vi "Create.vi"(8 "error in (no error)":errorcluster, 10 "Selected Group":T1, 11 "Chassis Link":T3) -> (0 "error out":errorcluster, 3 "Preview out":refnum<class "Preview.lvclass">)   [LabVIEW 2012, in "Preview Window.lvlib" / "Preview.lvclass"]
uses:
  Preview.lvclass
  Custom Ctrls/Master Cfg/ge_Cfg wChassis.ctl
  Cfg Grandmaster/Class Chassis BOM/Chassis BOM.lvclass
  Cfg Grandmaster/Class Chassis Cfg/ChassisCfg.lvclass
  Data Acquisition/Class Chassis Tasks/Chassis Tasks.lvclass
  Common/Controls/Selected Group.ctl
  Common/Controls/TE_Designator.ctl
  Preview.lvclass/Preview.ctl
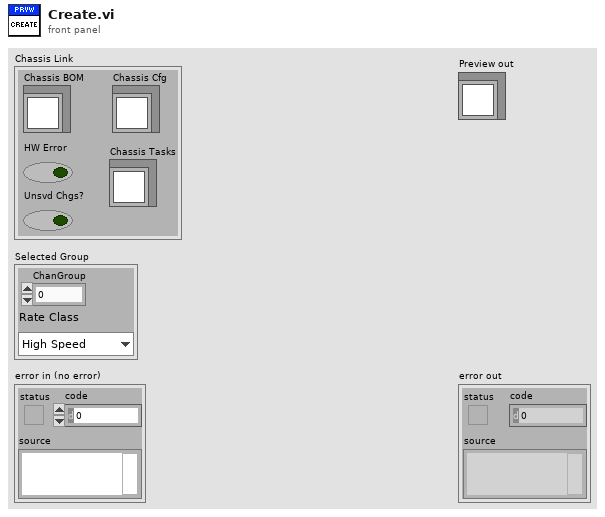
[diagram p1: front panel]
types:
  T1 = typedef "Selected Group.ctl" = cluster{"ChanGroup":i32, "Rate Class":T2}
  T2 = typedef "TE_Designator.ctl" = enum16{"High Speed", "Low Speed"}
  T3 = typedef "ge_Cfg wChassis.ctl" = cluster{"Chassis BOM":refnum<class "Chassis BOM.lvclass">, "Chassis Cfg":refnum<class "ChassisCfg.lvclass">, "Chassis Tasks":refnum<class "Chassis Tasks.lvclass">, "HW Error":bool, "Unsvd Chgs?":bool}
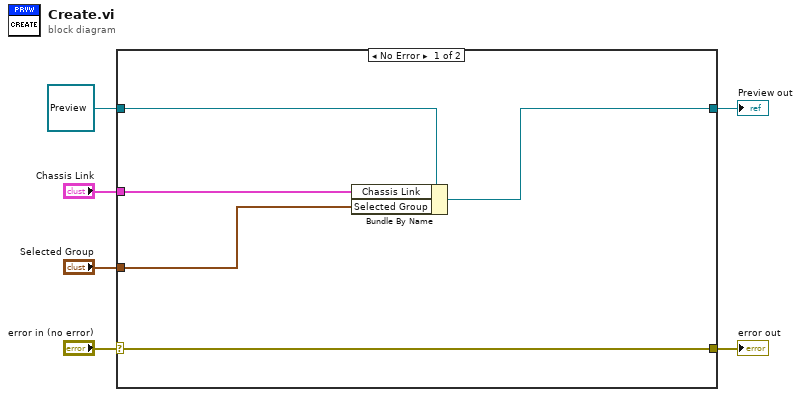
[diagram p0: block diagram]
diagram:
  n1 = case shown="No Error" "error in (no error)" {
    selector: "error in (no error)" -> [w11 w13]
    tunnel: [w11 w13] -> w5
    tunnel: [w9 w12] -> w3
    tunnel: refnum<class "Preview.lvclass"> refnum ("Preview in") -> [w10 w12]
    tunnel: "Chassis Link" -> [w8 _]
    tunnel: "Selected Group" -> [w7 _]
    frame No Error {
      n2 = Bundle By Name(cluster=w10, "Chassis Link"=w8, "Selected Group"=w7) -> (w9:refnum<class "Preview.lvclass">)
    }
    frame Error {
    }
  }
  "error out" <- w5
  "Preview out" <- w3
